vi "Twist_Equals.vi"(9 "other TWIST":T1, 11 "this TWIST":T1) -> (3 "Equals":bool)   [LabVIEW 2019, in "Trajectory_Library.lvlib"]
doc: "Checks equality between this Twist2d and another object.\n\nParameters:\n - this twist - This TWIST data structure\n - other twist - The other TWIST data structure to compare to\n\nReturns:\n - equals - Returns TRUE if both TWISTS are equal"
uses:
  Trajectory_Library.lvlib
  TWIST2D.ctl
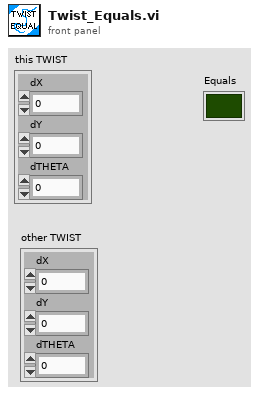
[diagram p1: front panel]
types:
  T1 = typedef "Trajectory_Library.lvlib/TWIST2D.ctl" = cluster{"dX":dbl, "dY":dbl, "dTHETA":dbl}
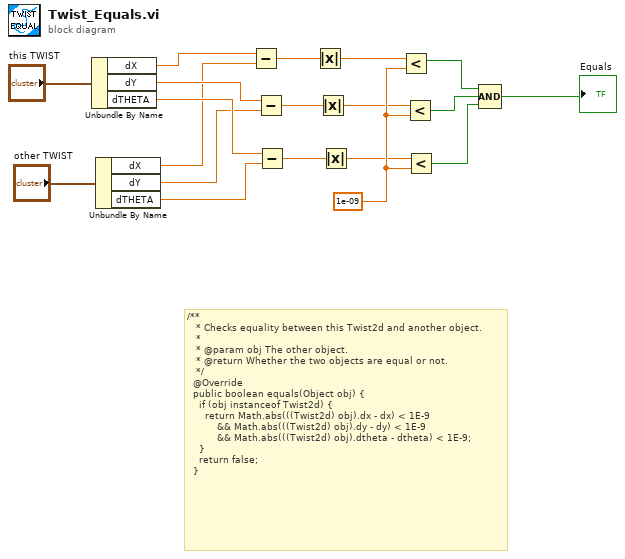
[diagram p0: block diagram]
diagram:
  w13 = 1e-09 ("y")
  # "/**\n   * Checks equality between this Twist2d and another object.\n   *\n   * @param obj The other object.\n   * @return Whether the two objects are equal or not.\n   */\n  @Override\n  public boolean equals(Object obj) {\n    if (obj instanceof Twist2d) {\n      return Math.abs(((Twist2d) obj).dx - dx) < 1E-9\n          && Math.abs(((Twist2d) obj).dy - dy) < 1E-9\n          && Math.abs(((Twist2d) obj).dtheta - dtheta) < 1E-9;\n    }\n    return false;\n  }"
  n1 = Unbundle By Name("this TWIST") -> ("dX"=w6:dbl, "dY"=w5:dbl, "dTHETA"=w4:dbl)
  n2 = Unbundle By Name("other TWIST") -> ("dX"=w3:dbl, "dY"=w2:dbl, "dTHETA"=w1:dbl)
  n3 = Subtract(x=w6, y=w3) -> (x-y=w9:dbl)
  n4 = Subtract(x=w5, y=w2) -> (x-y=w8:dbl)
  n5 = Subtract(x=w4, y=w1) -> (x-y=w7:dbl)
  n6 = Absolute Value(x=w9) -> (abs(x)=w12:dbl)
  n7 = Absolute Value(x=w8) -> (abs(x)=w11:dbl)
  n8 = Absolute Value(x=w7) -> (abs(x)=w10:dbl)
  n9 = Less?(x=w12, y=w13) -> (x < y?=w17:bool)
  n10 = Less?(x=w11, y=w13) -> (x < y?=w16:bool)
  n11 = Less?(x=w10, y=w13) -> (x < y?=w15:bool)
  n12 = Compound Arithmetic op=AND(w17, w16, w15) -> (→"Equals":bool)
